vi "scope_test1.vi"() -> ()   [LabVIEW 2023]
uses:
  Measure and Stimulus Subsystems/Measure and Stimulus Subsystems.lvclass
panel:
  out "Powersensor Chart":waveform(dbl)(graph)
  in  "Stop":bool
  out "Photosensor Chart":waveform(dbl)(graph)
  out "Error Out":errorcluster
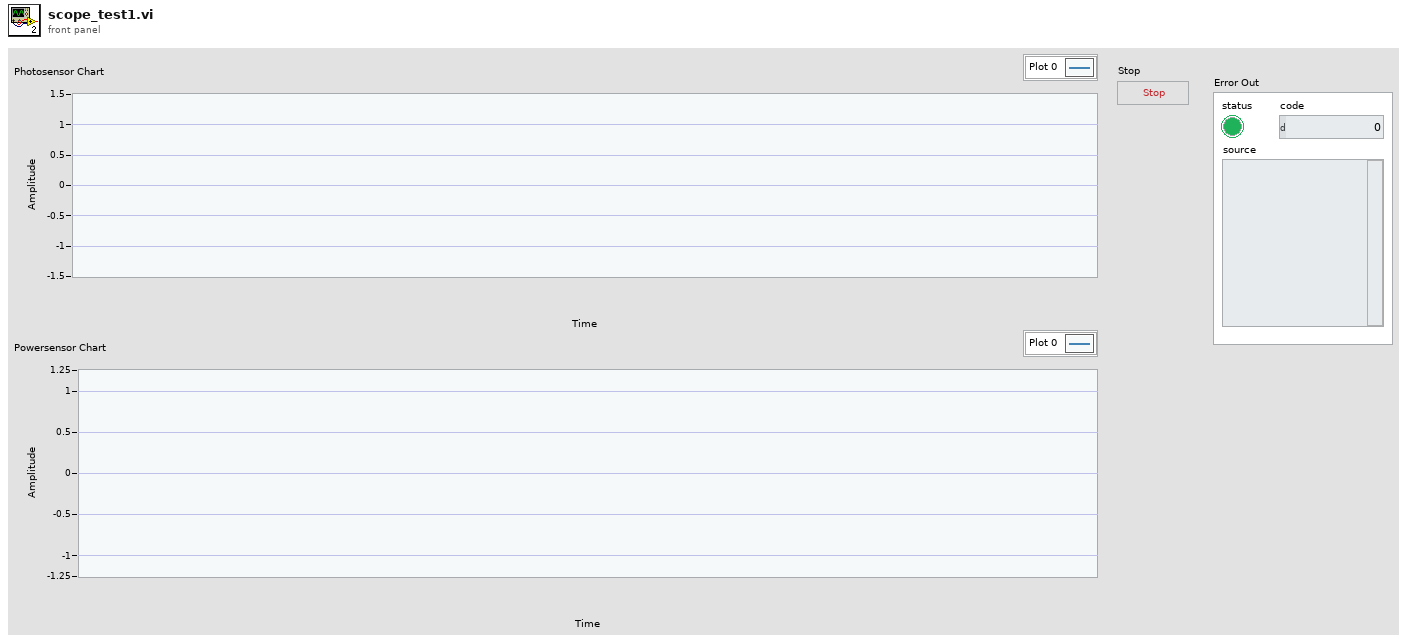
[diagram p1: front panel]
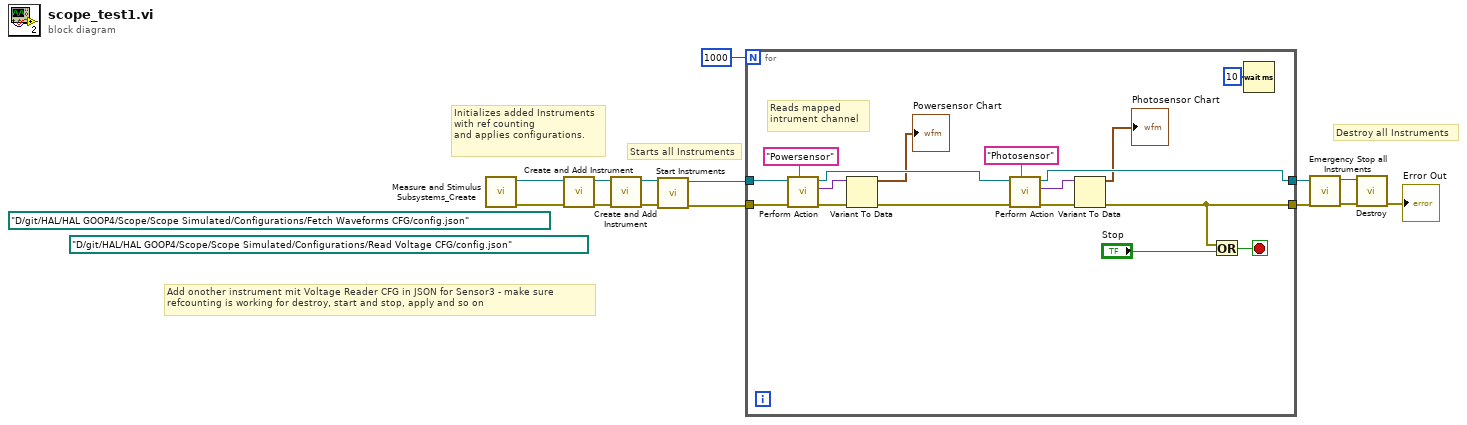
[diagram p0: block diagram]
diagram:
  (unwired) path "D:/git/HAL/HAL GOOP4/Scope/Scope Simulated/Configurations/Read Voltage CFG/config.json" ("File Path")
  (unwired) path "D:/git/HAL/HAL GOOP4/Scope/Scope Simulated/Configurations/Fetch Waveforms CFG/config.json" ("File Path")
  # "Add onother instrument mit Voltage Reader CFG in JSON for Sensor3 - make sure\nrefcounting is working for destroy, start and stop, apply and so on"
  # "Initializes added Instruments\nwith ref counting\nand applies configurations."
  # "Starts all Instruments"
  # "Destroy all Instruments"
  n1 = call "Measure and Stimulus Subsystems_Create.vi"() -> ("Error Out"=w13:errorcluster, "reference out"=w14:refnum<class "Measure and Stimulus Subsystems.lvclass">)  [unwired: 10 in]
  n2 = call-dynamic "Create and Add Instrument.vi"("Error In"=w13, "reference in"=w14) -> ("Error Out"=w4:errorcluster, "reference out"=w2:refnum<class "Measure and Stimulus Subsystems.lvclass">)  [unwired: 8 in]
  n3 = call-dynamic "Create and Add Instrument.vi"("Error In"=w4, "reference in"=w2) -> ("Error Out"=w3:errorcluster, "reference out"=w1:refnum<class "Measure and Stimulus Subsystems.lvclass">)  [unwired: 8 in]
  n4 = call "Start Instruments.vi"("Error In"=w3, "reference in"=w1) -> ("Error Out"=w6:errorcluster, "reference out"=w5:refnum<class "Measure and Stimulus Subsystems.lvclass">)  [unwired: 8 in]
  n5 = for {
    N: 1000 -> [_]
    tunnel: w6 -> [w23]
    tunnel: w5 -> [w22]
    tunnel: [w24] -> w10
    tunnel: [w26] -> w11
    stop <- w30 stop-if-true
    # "Reads mapped\nintrument channel"
    n6 = call "Perform Action.vi"("Target Ident"="Powersensor" ("Target Identifier"), "Error In"=w23, "reference in"=w22) -> ("Error Out"=w21:errorcluster, "Output"=w17:variant, "reference out"=w18:refnum<class "Measure and Stimulus Subsystems.lvclass">)  [unwired: 6 in]
    n7 = Variant To Data(error in=w21, Variant=w17) -> (data=→"Powersensor Chart":waveform(dbl), error out=w19:errorcluster)  [unwired: 1 in]
    n8 = call "Perform Action.vi"("Target Ident"="Photosensor" ("Target Identifier"), "Error In"=w19, "reference in"=w18) -> ("Error Out"=w28:errorcluster, "Output"=w25:variant, "reference out"=w24:refnum<class "Measure and Stimulus Subsystems.lvclass">)  [unwired: 6 in]
    n9 = Variant To Data(error in=w28, Variant=w25) -> (data=→"Photosensor Chart":waveform(dbl), error out=w26:errorcluster)  [unwired: 1 in]
    n10 = Or(x=w26, y="Stop") -> (x .or. y?=w30:bool)
    n11 = Wait (ms)(milliseconds to wait=u32 10) -> ()  [unwired: 1 out]
  }
  n12 = call "Emergency Stop all Instruments.vi"("Error In"=w11, "reference in"=w10) -> ("Error Out"=w9:errorcluster, "reference out"=w8:refnum<class "Measure and Stimulus Subsystems.lvclass">)  [unwired: 8 in]
  n13 = call-dynamic "Destroy.vi"("Error In"=w9, "reference in"=w8) -> ("Error Out"=→"Error Out":errorcluster)  [unwired: 8 in, 1 out]
